vi "Control Data Viewer.vi"() -> ()   [LabVIEW 2018]
uses:
  user32.dll
panel:
  in  "Abort":bool
  in  "Title Bar":bool caption="Blank"
  in  "Load File":bool caption="Open"
  out "Esforços de controle":waveform(dbl)[](graph)
  out "Níveis dos Tanques":waveform(dbl)[](graph)
  # "Controle Robusto - Tanque quádruplo"
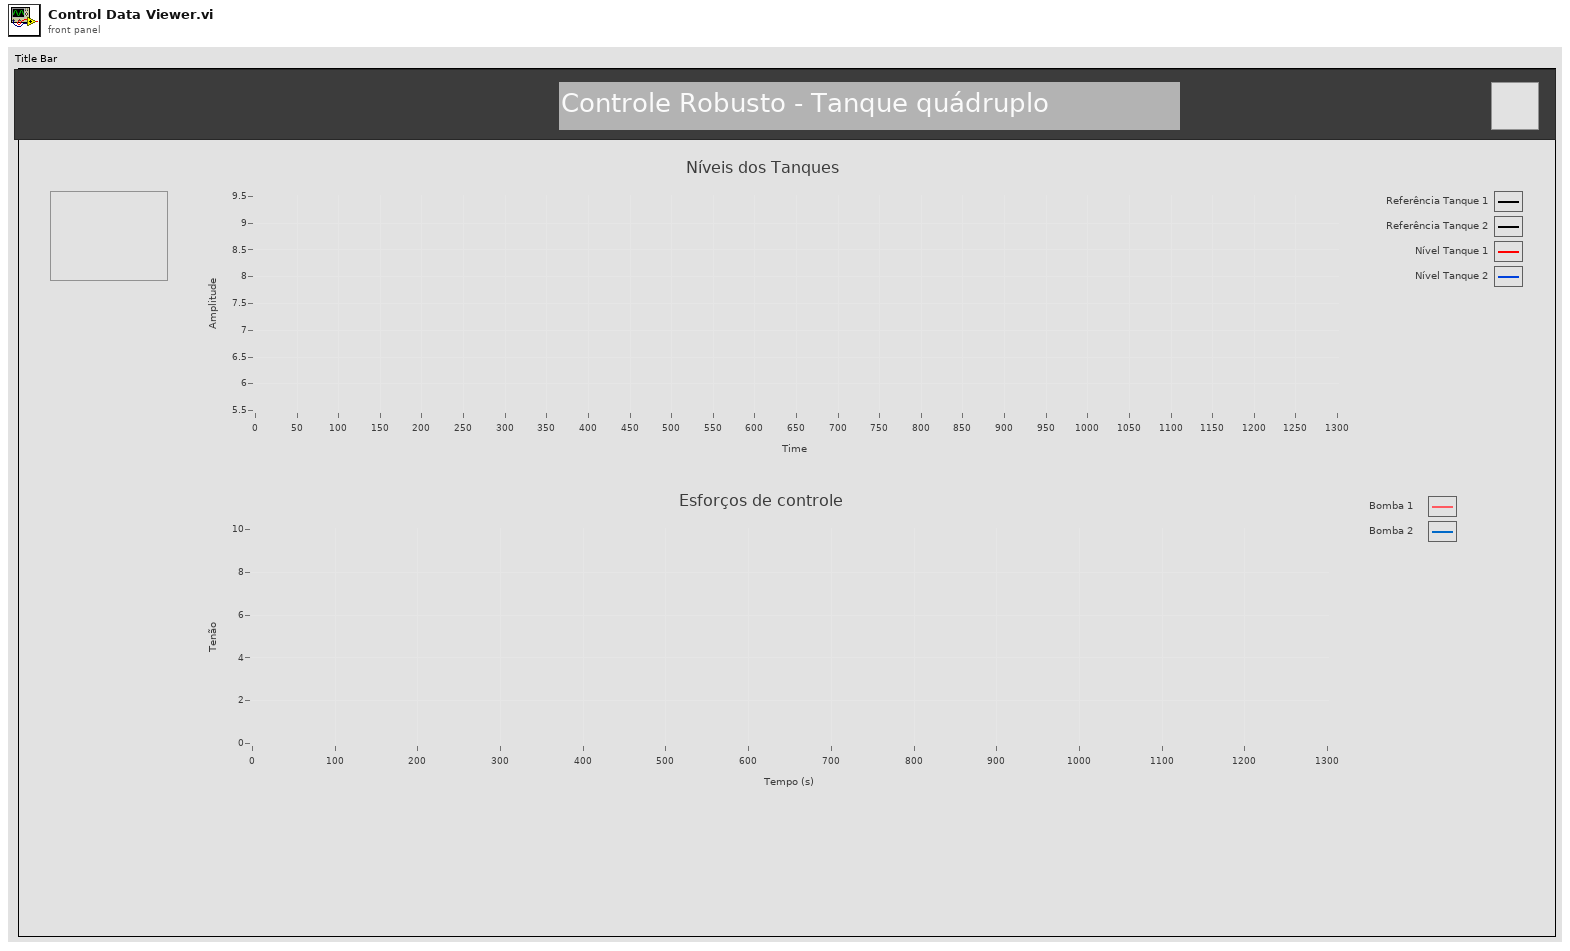
[diagram p1: front panel]
types:
  T1 = enum16{"open", "open or create", "create or replace", "create", "open (read-only)"}
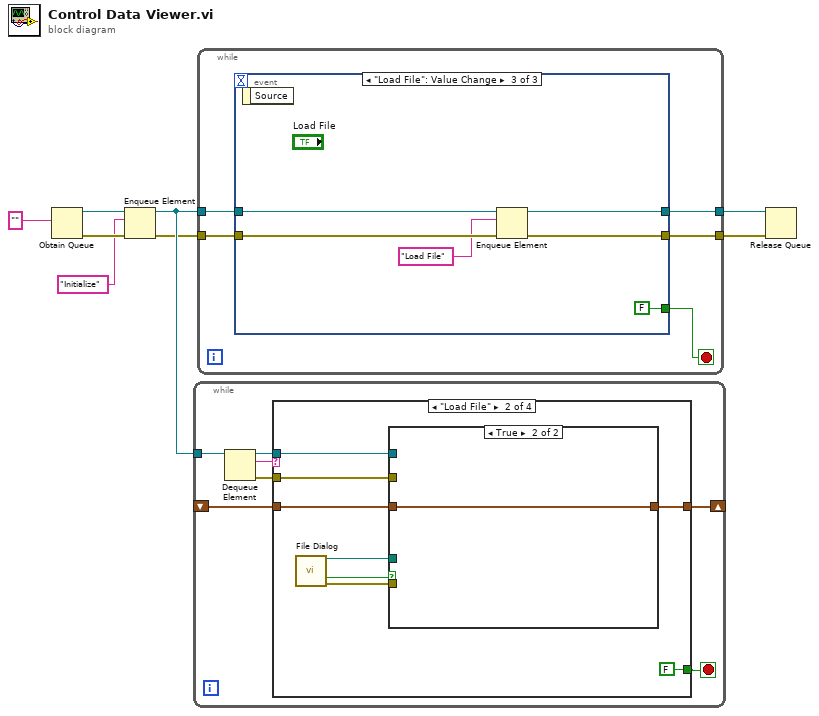
[diagram p0: block diagram]
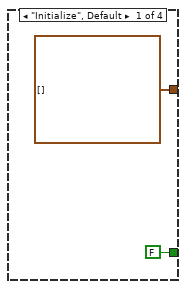
[diagram p2: hidden frame]
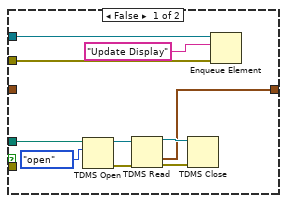
[diagram p3: hidden frame]
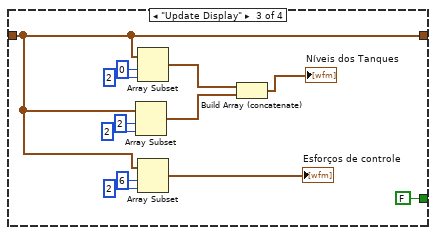
[diagram p4: hidden frame]
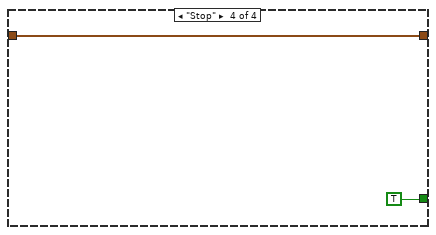
[diagram p5: hidden frame]
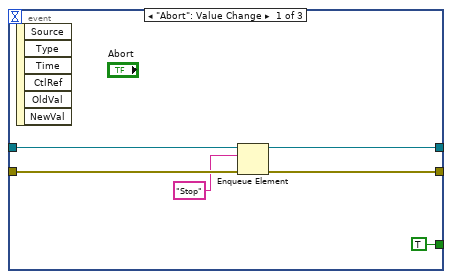
[diagram p6: hidden frame]
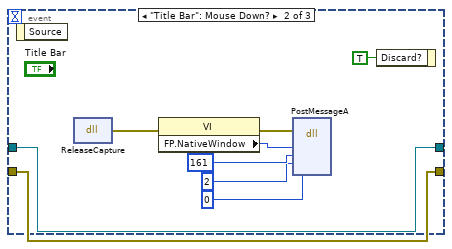
[diagram p7: hidden frame]
diagram:
  n1 = Obtain Queue(element data type="" ("element")) -> (queue out=w6:refnum<queue>, error out=w4:errorcluster)  [unwired: 4 in, 1 out]
  n2 = Enqueue Element(queue=w6, element="Initialize", error in (no error)=w4) -> (queue out=w5:refnum<queue>, error out=w3:errorcluster)  [unwired: 1 in, 1 out]
  n3 = while {
    tunnel: w5 -> [w15]
    shift-right: [w11] -> _
    shift-left: _ -> [w10]
    stop <- w12 stop-if-true
    n4 = Dequeue Element(queue=w15) -> (queue out=w13:refnum<queue>, element=w14:string, error out=w9:errorcluster)  [unwired: 2 in, 1 out]
    n5 = case shown="\"Load File\"" w14 {
      tunnel: w13 -> [_ w25 _ _]
      tunnel: [FALSE FALSE FALSE TRUE] -> w12
      tunnel: [waveform(dbl)[] [] ("data") w23 w37 w49] -> w11
      tunnel: w10 -> [_ w20 w37 w49]
      tunnel: w9 -> [_ w19 _ _]
      frame "Initialize", Default {
      }
      frame "Load File" {
        n6 = call "File Dialog"() -> ("selected path"=w22:path, "cancelled"=w21:bool, "error out"=w18:errorcluster)  [unwired: 12 in, 1 out]
        n7 = case shown="True" w21 {
          tunnel: w25 -> [w34 _]
          tunnel: [w28 w36] -> w23
          tunnel: w22 -> [w27 _]
          tunnel: w20 -> [_ w36]
          tunnel: w19 -> [w26 _]
          tunnel: w18 -> [_ _]
          frame False {
            n8 = TDMS Open(10:T1."open" ("operation (0:open)"), 11:w27) -> (0:w32:errorcluster, 3:w33:refnum<k34>)  [unwired: 5 in]
            n9 = TDMS Read(0:w33, 11:w32) -> (4:w31:refnum<k34>, 10:w28:waveform(dbl)[], 15:w30:errorcluster)  [unwired: 6 in, 3 out]
            n10 = TDMS Close(8:w30, 11:w31) -> ()  [unwired: 2 out]
            n11 = Enqueue Element(queue=w34, element="Update Display", error in (no error)=w26) -> ()  [unwired: 1 in, 3 out]
          }
          frame True {
          }
        }
      }
      frame "Update Display" {
        n12 = Array Subset(array=w37, index=2, length=2) -> (w46:waveform(dbl)[])
        n13 = Array Subset(array=w37, index=0, length=2) -> (w44:waveform(dbl)[])
        n14 = Array Subset(array=w37, index=6, length=2) -> (→"Esforços de controle":waveform(dbl)[])
        n15 = Build Array (concatenate)(w44, w46) -> (→"Níveis dos Tanques":waveform(dbl)[])
      }
      frame "Stop" {
      }
    }
  }
  n16 = while {
    tunnel: w5 -> [w55]
    tunnel: [w54] -> w8
    tunnel: w3 -> [w53]
    tunnel: [w52] -> w7
    stop <- w51 stop-if-true
    n17 = event shown="[2] \"Load File\": Value Change" {
      selector: _ -> [_ _ _]
      dyn-events: _ -> [_ _ _]
      timeout: _ -> [_ _ _]
      tunnel: w55 -> [w61 w68 w76]
      tunnel: [w60 w68 w75] -> w54
      tunnel: w53 -> [w59 w69 w74]
      tunnel: [w58 w69 w73] -> w52
      tunnel: [TRUE _ FALSE] -> w51
      event "Abort": Value Change {
        n18 = event-data() -> ()  [unwired: 1 in, 6 out]
        n19 = Enqueue Element(queue=w61, element="Stop", error in (no error)=w59) -> (queue out=w60:refnum<queue>, error out=w58:errorcluster)  [unwired: 1 in, 1 out]
      }
      event "Title Bar": Mouse Down? {
        n20 = event-data() -> ()  [unwired: 1 in, 1 out]
        n21 = dll-call lib="user32.dll" fn="ReleaseCapture"() -> (error out=w65:errorcluster)  [unwired: 4 in, 1 out]
        n22 = property class="VI"(error in=w65) -> (error out=w66:errorcluster, "FP.NativeWindow"=w67:u64)  [unwired: 1 in, 1 out]
        n23 = dll-call lib="user32.dll" fn="PostMessageA"(error in=w66, "hWnd"=w67, "Msg"=161, "wParam"=2, "lParam"=0) -> ()  [unwired: 7 in, 2 out]
        n24 = event-data("Discard?"=TRUE) -> ()  [unwired: 1 in, 1 out]
      }
      event "Load File": Value Change {
        n25 = event-data() -> ()  [unwired: 1 in, 1 out]
        n26 = Enqueue Element(queue=w76, element="Load File", error in (no error)=w74) -> (queue out=w75:refnum<queue>, error out=w73:errorcluster)  [unwired: 1 in, 1 out]
      }
    }
  }
  n27 = Release Queue(queue=w8, error in (no error)=w7) -> ()  [unwired: 1 in, 3 out]
